vi "_Clear Parent.vi"(8 "error in (no error)":errorcluster, 11 "NodeRef In":refnum<data-value>) -> (0 "error out":errorcluster, 3 "NodeRef":refnum<data-value>)   [LabVIEW 2020, in "PicoG-ParserLexer.lvlib" / "Node.lvclass"]
uses:
  Node.lvclass
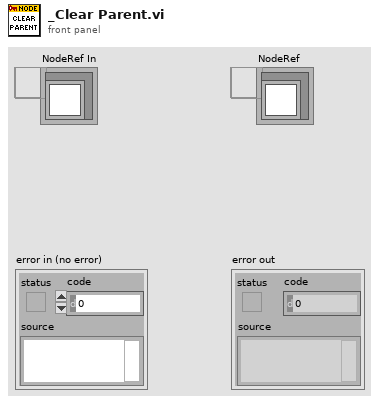
[diagram p1: front panel]
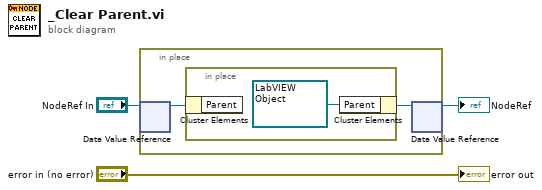
[diagram p0: block diagram]
diagram:
  n1 = in-place {
    n2 = in-place-dvr #1("NodeRef In") -> (w5:refnum<class "Node.lvclass">)  [unwired: 1 out]
    n3 = in-place {
      n4 = in-place-cluster #2(w5) -> ()  [unwired: 1 out]
      n5 = in-place-cluster #2("Parent"=refnum<data-value> refnum) -> (w4:refnum<class "Node.lvclass">)
    }
    n6 = in-place-dvr #1(w4) -> (→"NodeRef":refnum<data-value>)  [unwired: 1 out]
  }
  "error out" <- "error in (no error)"
